vi "Automatically Zero Input.vi"(8 "error in (no error)":errorcluster, 10 "Channel":T1, 11 "EPU452 in":refnum<class "EPU452.lvclass">) -> (0 "error out":errorcluster, 2 "Response":string, 3 "EPU452 out":refnum<class "EPU452.lvclass">)   [LabVIEW 2018, in "EPU452.lvclass"]
uses:
  EPU452.lvclass
  Controls/Channels.ctl
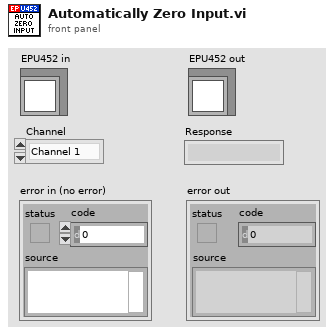
[diagram p1: front panel]
types:
  T1 = typedef "EPU452.lvclass/Channels.ctl" = enum16{"Channel 1", "Channel 2", "Channel 3", "Channel 4"}
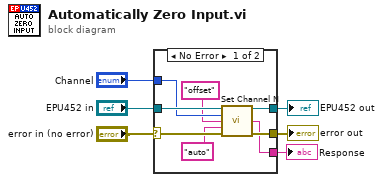
[diagram p0: block diagram]
diagram:
  n1 = case shown="No Error" "error in (no error)" {
    selector: "error in (no error)" -> [w11 w16]
    tunnel: [w8 w16] -> w5
    tunnel: [w9 w15] -> w3
    tunnel: "EPU452 in" -> [w14 w15]
    tunnel: "Channel" -> [w13 _]
    tunnel: [w7 _] -> w1
    frame No Error {
      n2 = call "Set Channel N.vi"("EPU452 in"=w14, "Channel"=w13, "Function"="offset", "Argument/s"="auto", "error in (no error)"=w11) -> ("EPU452 out"=w9:refnum<class "EPU452.lvclass">, "Response"=w7:string, "error out"=w8:errorcluster)  [unwired: 8 in]
    }
    frame Error {
    }
  }
  "error out" <- w5
  "EPU452 out" <- w3
  "Response" <- w1
